vi "ThorOCT Spatial Trim.vi"(7 "#pixels to save":i32=300, 8 "error in":errorcluster, 9 "start pixel":i32, 10 "#A-lines":i32=2048, 11 "2D Array in":sgl[][](array[numeric])) -> (0 "error out":errorcluster, 3 "array for saving":sgl[](array[numeric]))   [LabVIEW 2018]
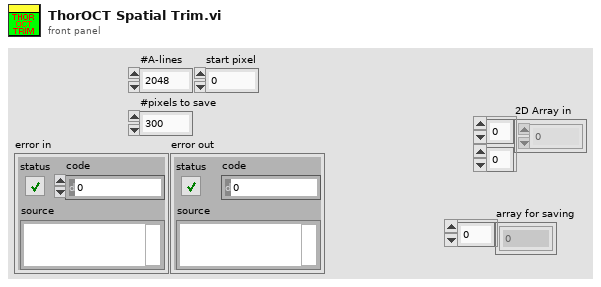
[diagram p1: front panel]
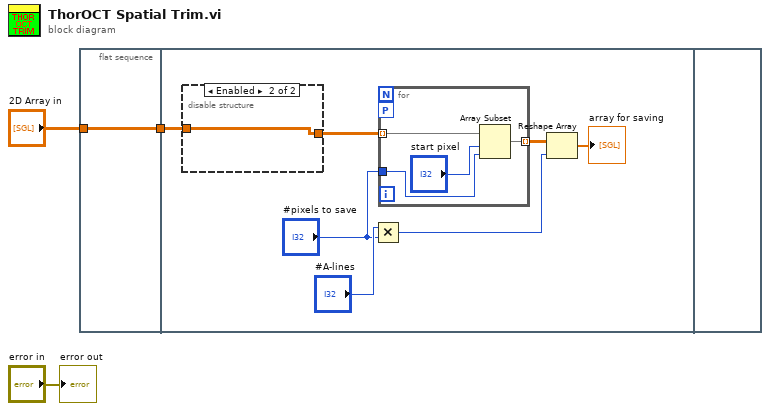
[diagram p0: block diagram]
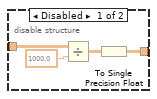
[diagram p2: hidden frame]
diagram:
  n1 = flat-sequence {
    tunnel: "2D Array in" -> [w4]
    tunnel: [w4] -> w3
    tunnel: w3 -> [w11]
    frame #0 {
    }
    frame #1 {
      n2 = disable-structure shown="Enabled" {
        disable-tunnel: w11 -> [w19 w20]
        disable-tunnel: [w16 w20] -> w10
        frame Disabled {
          n3 = Divide(x=w19, y=sgl 1000.0) -> (x/y=w17:sgl[][])
          n4 = To Single Precision Float(number=w17) -> (single precision float=w16:sgl[][])
        }
        frame Enabled {
        }
      }
      n5 = Multiply(x="#A-lines", y="#pixels to save") -> (x*y=w6:i32)
      n6 = for {
        tunnel: w10 -> [w15] mode=indexing
        workers-P: _ -> [_]
        tunnel: [w14] -> w9 mode=indexing
        tunnel: "#pixels to save" -> [w13]
        n7 = Array Subset(array=w15, index="start pixel", length=w13) -> (w14:sgl[])
      }
      n8 = Reshape Array(w9, w6) -> (→"array for saving":sgl[])
    }
    frame #2 {
    }
  }
  "error out" <- "error in"
